vi "read ids.vi"(8 "error in (no error)":errorcluster) -> (0 "error out":errorcluster, 3 "ids":string[](array[string]))   [LabVIEW 2024, in "controls manager.lvlib"]
uses:
  controls manager.lvlib
  fgv actions.ctl
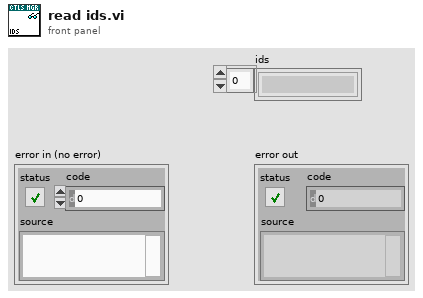
[diagram p1: front panel]
types:
  T1 = typedef "controls manager.lvlib/fgv actions.ctl" = enum16{"create", "get", "destroy"}
  T2 = typedef "controls manager.lvlib/collection type.ctl" = map{string, T3}
  T3 = typedef "controls manager.lvlib/entry type.ctl" = cluster{"controls":map{string, T4}, "plan":T5}
  T4 = typedef "controls manager.lvlib/control.ctl" = cluster{"refnum":refnum<vi>, "index":i32}
  T5 = typedef "controls manager.lvlib/controls plan.ctl" = map{string, T6[]}
  T6 = typedef "controls manager.lvlib/key value pair.ctl" = cluster{"key":string, "value":string}
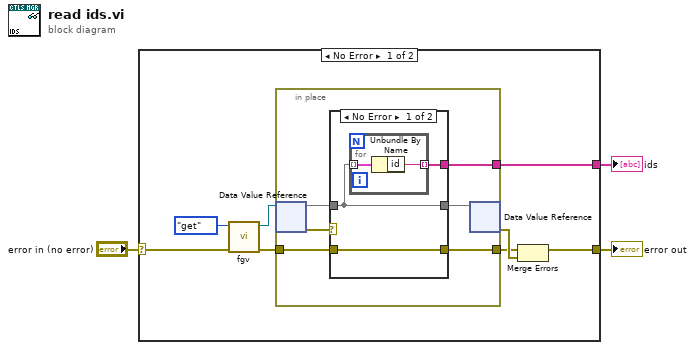
[diagram p0: block diagram]
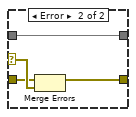
[diagram p2: hidden frame]
diagram:
  n1 = case shown="No Error" "error in (no error)" {
    selector: "error in (no error)" -> [w7 w27]
    tunnel: [w9 w27] -> w2
    tunnel: [w4 _] -> w1
    frame No Error {
      n2 = call "fgv.vi"("error in (no error)"=w7, "action"=fgv_actions."get") -> ("error out"=w6:errorcluster, "dvr"=w8:refnum<data-value>)  [unwired: 8 in]
      n3 = in-place {
        in-place-border: w6 -> [w15]
        in-place-border: [w14] -> w10
        in-place-border: [w12] -> w4
        n4 = in-place-dvr #1(w8) -> (w17:T2, w13:errorcluster)
        n5 = case shown="No Error" w13 {
          selector: w13 -> [_ w25]
          tunnel: w17 -> [w20 w26]
          tunnel: [w20 w26] -> w16
          tunnel: w15 -> [w19 w24]
          tunnel: [w19 w23] -> w14
          tunnel: [w18 _] -> w12
          frame No Error {
            n6 = for {
              tunnel: w20 -> [w22] mode=indexing
              tunnel: [w21] -> w18 mode=indexing
              n7 = Unbundle By Name(w22) -> ("id"=w21:string)
            }
          }
          frame Error {
            n8 = Merge Errors(w24, w25) -> (w23:errorcluster)
          }
        }
        n9 = in-place-dvr #1(w16) -> (w11:errorcluster)  [unwired: 1 out]
      }
      n10 = Merge Errors(w10, w11) -> (w9:errorcluster)
    }
    frame Error {
    }
  }
  "error out" <- w2
  "ids" <- w1
